vi "Write Initialized.vi"(8 "error in (no error)":errorcluster, 10 "Initialized":bool, 11 "DDS in":refnum<class "DDS.lvclass">) -> (0 "error out":errorcluster, 3 "DDS out":refnum<class "DDS.lvclass">)   [LabVIEW 2013, in "DDS.lvclass"]
uses:
  DDS.lvclass
  DDS.lvclass/DDS.ctl
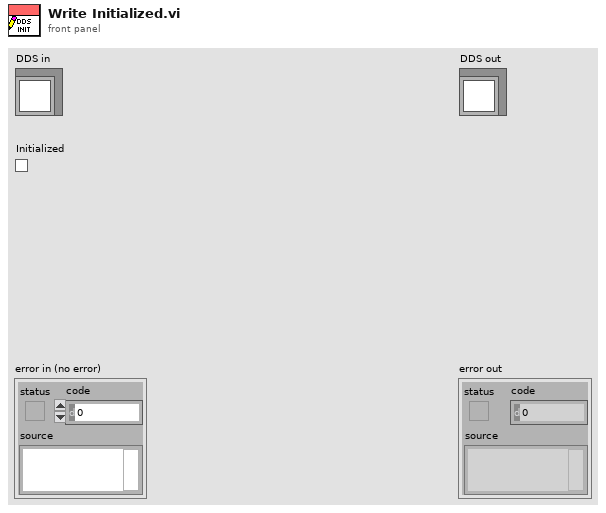
[diagram p1: front panel]
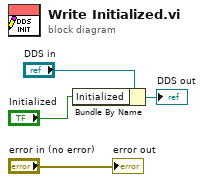
[diagram p0: block diagram]
diagram:
  n1 = Bundle By Name(cluster="DDS in", "Initialized"="Initialized") -> (→"DDS out":refnum<class "DDS.lvclass">)
  "error out" <- "error in (no error)"
